vi "SetErrorMessage.vi"(8 "error in (no error)":errorcluster, 9 "Error Message":string, 10 "Tag Name":string, 11 "ResultTree in":refnum<class "ResultTree.lvclass">) -> (0 "error out":errorcluster, 3 "ResultTree out":refnum<class "ResultTree.lvclass">)   [LabVIEW 2019, in "ResultTree.lvclass"]
doc: "Sets the error message."
uses:
  ResultTree.lvclass
  ResultTree.lvclass/ResultTree.ctl
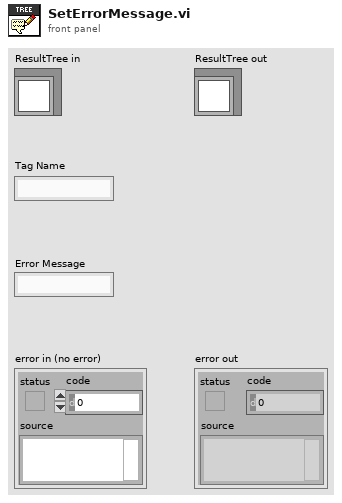
[diagram p1: front panel]
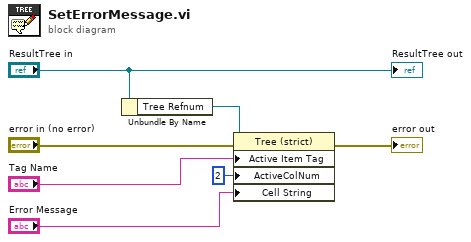
[diagram p0: block diagram]
diagram:
  n1 = Unbundle By Name("ResultTree in") -> ("Tree Refnum"=w4:refnum<vi>)
  n2 = property class="Tree (strict)"(reference=w4, error in="error in (no error)", "Active Item Tag"="Tag Name", "ActiveColNum"=2 ("Active Cell:Active Column Number"), "Cell String"="Error Message") -> (error out=→"error out":errorcluster)  [unwired: 1 out]
  "ResultTree out" <- "ResultTree in"
